vi "libzmq path.vi"() -> (2 "path":path)   [LabVIEW 2019, in "RemoteControl.ZMQ.lvlib" / "libzmq.lvclass"]
uses:
  libzmq.lvclass
  libzmq32/libzmq32.lvclass
  libzmq64/libzmq64.lvclass
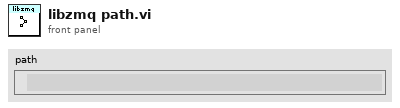
[diagram p1: front panel]
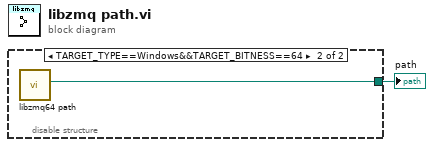
[diagram p0: block diagram]
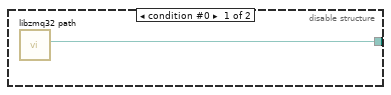
[diagram p2: hidden frame]
diagram:
  n1 = disable-structure shown="TARGET_TYPE==Windows&&TARGET_BITNESS==64" {
    disable-tunnel: [w2 w3] -> w1
    frame condition #0 {
      n2 = call "libzmq32 path.vi"() -> ("path"=w2:path)  [unwired: 11 in]
    }
    frame condition #1 (active) {
      n3 = call "libzmq64 path.vi"() -> ("path"=w3:path)  [unwired: 11 in]
    }
  }
  "path" <- w1
